vi "test Message - Put Get Delete.vi"(8 "error in (no error)":errorcluster, 11 "TestCase in":refnum<class "Test_Queue.lvclass">) -> (0 "error out":errorcluster, 3 "TestCase out":refnum<class "Test_Queue.lvclass">)   [LabVIEW 2015, in "Test_Queue.lvclass"]
uses:
  Test_Queue.lvclass
  Global Parameters.vi
  Core/Session/Session.lvclass
  Queue/NI_Azure_Queue.lvlib
  _shared/_Unit Tests Shared.lvlib
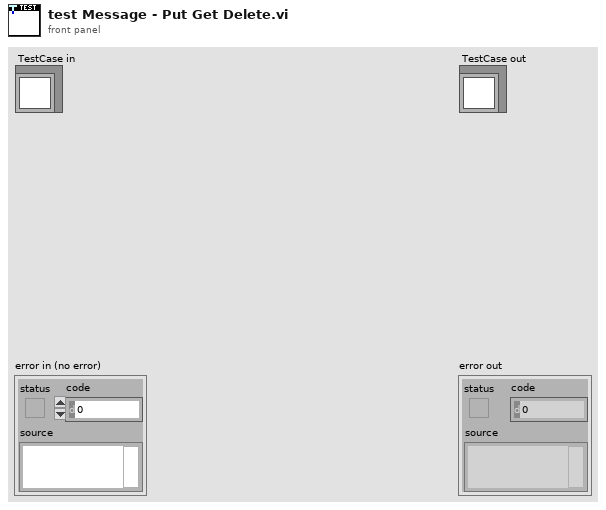
[diagram p1: front panel]
types:
  T1 = typedef "NI_Azure_Core.lvlib/Azure Credentials.ctl" = cluster{"Storage Account Name":string, "Access Key":string}
  T2 = typedef "NI_Azure_Queue.lvlib/Message.ctl" = cluster{"Message ID":string, "Insertion Time":string, "Expiration Time":string, "Pop Receipt":string, "Time Next Visible":string, "Dequeue Count":i32, "Message Text":string}
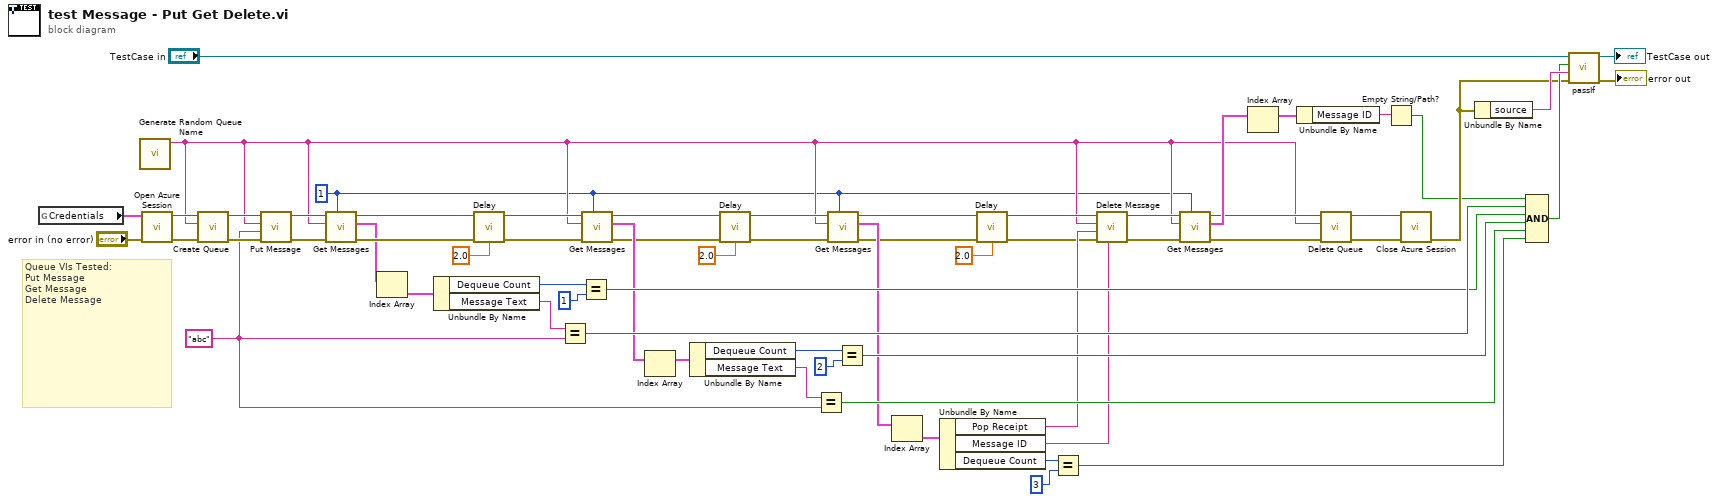
[diagram p0: block diagram]
diagram:
  w4 = u32 1 ("Visibility timeout (30 seconds)")
  w32 = "abc" ("Message")
  # "Queue VIs Tested:\nPut Message\nGet Message\nDelete Message"
  n1 = global read "Global Parameters.vi" "Credentials"() -> (w54:T1)
  n2 = call "Generate Random Queue Name.vi"() -> ("Random Queue Name"=w18:string)  [unwired: 11 in]
  n3 = call "Open Azure Session.vi"("error in (no error)"="error in (no error)", "Credentials"=w54) -> ("error out"=w55:errorcluster, "Azure Session"=w50:refnum<class "Session.lvclass">)  [unwired: 8 in]
  n4 = call "Create Queue.vi"("error in (no error)"=w55, "Queue"=w18, "Azure Session in"=w50) -> ("error out"=w51:errorcluster, "Azure Session out"=w46:refnum<class "Session.lvclass">)  [unwired: 7 in]
  n5 = call "Put Message.vi"("error in (no error)"=w51, "Message"=w32, "Queue"=w18, "Azure Session in"=w46) -> ("error out"=w47:errorcluster, "Azure Session out"=w45:refnum<class "Session.lvclass">)  [unwired: 5 in, 1 out]
  n6 = call "Get Messages.vi"("Visibility timeout (30 seconds)"=w4, "error in (no error)"=w47, "Queue"=w18, "Azure Session in"=w45) -> ("error out"=w16:errorcluster, "Messages"=w10:T2[], "Azure Session out"=w35:refnum<class "Session.lvclass">)  [unwired: 5 in]
  n7 = Index Array(array=w10) -> (element=w9:T2)  [unwired: 1 in]
  n8 = Unbundle By Name(w9) -> ("Dequeue Count"=w42:i32, "Message Text"=w44:string)
  n9 = call "Delay.vi"("error in"=w16, "delay (1 sec)"=2.0) -> ("error out"=w15:errorcluster)  [unwired: 13 in]
  n10 = Equal?(x=w44, y=w32) -> (x = y?=w43:bool)
  n11 = Equal?(x=w42, y=1) -> (x = y?=w40:bool)
  n12 = call "Get Messages.vi"("Visibility timeout (30 seconds)"=w4, "error in (no error)"=w15, "Queue"=w18, "Azure Session in"=w35) -> ("error out"=w2:errorcluster, "Messages"=w36:T2[], "Azure Session out"=w31:refnum<class "Session.lvclass">)  [unwired: 5 in]
  n13 = Index Array(array=w36) -> (element=w8:T2)  [unwired: 1 in]
  n14 = Unbundle By Name(w8) -> ("Dequeue Count"=w38:i32, "Message Text"=w37:string)
  n15 = call "Delay.vi"("error in"=w2, "delay (1 sec)"=2.0) -> ("error out"=w1:errorcluster)  [unwired: 13 in]
  n16 = Equal?(x=w37, y=w32) -> (x = y?=w33:bool)
  n17 = call "Get Messages.vi"("Visibility timeout (30 seconds)"=w4, "error in (no error)"=w1, "Queue"=w18, "Azure Session in"=w31) -> ("error out"=w12:errorcluster, "Messages"=w28:T2[], "Azure Session out"=w26:refnum<class "Session.lvclass">)  [unwired: 5 in]
  n18 = Equal?(x=w38, y=2) -> (x = y?=w34:bool)
  n19 = Index Array(array=w28) -> (element=w7:T2)  [unwired: 1 in]
  n20 = Unbundle By Name(w7) -> ("Pop Receipt"=w17:string, "Message ID"=w5:string, "Dequeue Count"=w29:i32)
  n21 = call "Delay.vi"("error in"=w12, "delay (1 sec)"=2.0) -> ("error out"=w11:errorcluster)  [unwired: 13 in]
  n22 = Equal?(x=w29, y=3) -> (x = y?=w27:bool)
  n23 = call "Delete Message.vi"("Message ID"=w5, "error in (no error)"=w11, "Pop Receipt"=w17, "Queue"=w18, "Azure Session in"=w26) -> ("error out"=w25:errorcluster, "Azure Session out"=w24:refnum<class "Session.lvclass">)  [unwired: 5 in]
  n24 = call "Get Messages.vi"("Visibility timeout (30 seconds)"=w4, "error in (no error)"=w25, "Queue"=w18, "Azure Session in"=w24) -> ("error out"=w19:errorcluster, "Messages"=w23:T2[], "Azure Session out"=w20:refnum<class "Session.lvclass">)  [unwired: 5 in]
  n25 = Index Array(array=w23) -> (element=w6:T2)  [unwired: 1 in]
  n26 = Unbundle By Name(w6) -> ("Message ID"=w22:string)
  n27 = call "Delete Queue.vi"("error in (no error)"=w19, "Queue"=w18, "Azure Session in"=w20) -> ("error out"=w49:errorcluster, "Azure Session out"=w48:refnum<class "Session.lvclass">)  [unwired: 7 in]
  n28 = Empty String/Path?(string/path=w22) -> (empty?=w21:bool)
  n29 = call "Close Azure Session.vi"("error in (no error)"=w49, "Azure Session"=w48) -> ("error out"=w52:errorcluster)  [unwired: 9 in]
  n30 = Unbundle By Name(w52) -> ("source"=w57:string)
  n31 = Compound Arithmetic op=AND(w21, w43, w40, w34, w33, w27) -> (w53:bool)
  n32 = call-dynamic "passIf.vi"("error in (no error)"=w52, "message (\"\")"=w57, "pass"=w53, "TestCase in"="TestCase in") -> ("error out"=→"error out":errorcluster, "TestCase out"=→"TestCase out":refnum<class "Test_Queue.lvclass">)  [unwired: 6 in]
